vi "VNS Zobolas Local Search wOSSPClass.vi"(0 "OSSP_Problem.lvclass":refnum<class "OSSP_Problem.lvclass">, 1 "Max Allowed Time Passed?":bool, 3 "Reorder?":bool, 5 "Schedule In":u16[](array[numeric]), 7 "Scheduler":T1, 9 "Max Iteration Count":i32=1, 11 "error in (no error)":errorcluster, 12 "Number of Neighborhoods":i32=2, 14 "Objective":T2) -> (4 "OSSP_Problem out":refnum<class "OSSP_Problem.lvclass">, 6 "VNS Result Out":u16[](array[numeric]), 10 "Makespan/Tardiness(FIFO Engine)":u16, 15 "error out":errorcluster)   [LabVIEW 2013]
uses:
  Classes/OSSP_Problem.lvclass
  GA/Controls/Objective.ctl
  GA/Controls/Scheduler Type.ctl
  Classes/OSSP_Problem.lvclass/OSSP_Problem.ctl
  GA/SubVIS/Remove Duplicates In Array.vi
  Generate Two Indices for Local Search.vi
  Or-Opt(Zobolas) Neighborhood.vi
  Classes/Scheduler_Class/Prins FIFO Scheduler Methods and Controls/Methods/Calculate Makespan (Prins FIFO Engine).vi
  Classes/Scheduler_Class/Prins FIFO Scheduler Methods and Controls/Methods/Calculate Tardiness (Prins FIFO Engine).vi
  Classes/Scheduler_Class/NonDelay Scheduler/Non Delay Scheduler Engine.vi
  Classes/OSSP_Problem_Class/Getters/Read Number of Jobs.vi
  Classes/OSSP_Problem_Class/Getters/Read Processing Times.vi
  GA/SubVIS/Calcualte General Tardiness.vi
  Classes/OSSP_Problem_Class/Getters/Read Due Dates.vi
  Classes/Scheduler_Class/Giffler Thompson Active Schedule Engine.vi
  Classes/Scheduler_Class/Prins FIFO Scheduler Methods and Controls/Prins FIFO Scheduler.vi
  Classes/Scheduler_Class/Prins FIFO Scheduler Methods and Controls/Methods/Calculate Final Completion Times of Jobs.vi
  Classes/Scheduler_Class/Prins FIFO Scheduler Methods and Controls/Methods/Reorder Schedule(Prins FIFO) based on Start Times.vi
  Classes/Scheduler_Class/Operation to Machine Job Tuple.vi
  Classes/Scheduler_Class/Prins FIFO Scheduler Methods and Controls/Methods/UpdateMachineGaps.vi
  Classes/Scheduler_Class/Prins FIFO Scheduler Methods and Controls/Methods/UpdateJobGaps.vi
  Classes/Scheduler_Class/Prins FIFO Scheduler Methods and Controls/Methods/Find Intersecting Gaps.vi
  Classes/Scheduler_Class/GT Algorithm Find M_ok and J_ok.vi
  Classes/Scheduler_Class/Prins FIFO Scheduler Methods and Controls/Methods/Transform to Plain Job and Machine Gaps Array.vi
  Classes/Scheduler_Class/Semiactive Scheduler/Semi Active Scheduler Engine.vi
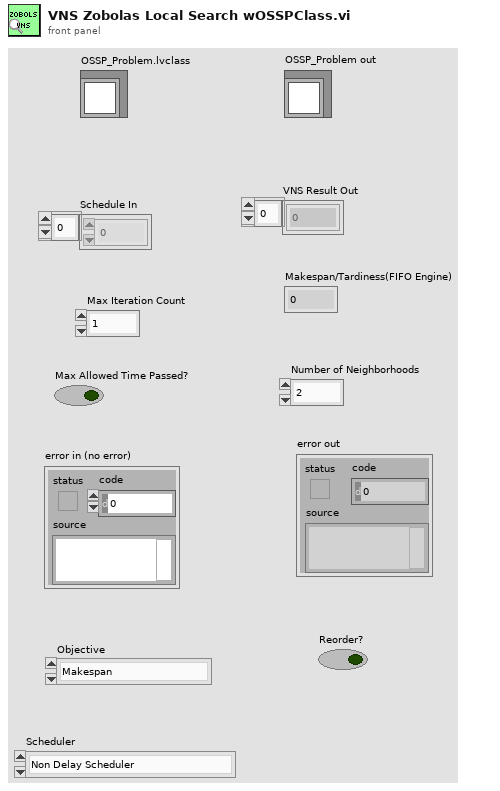
[diagram p1: front panel]
types:
  T1 = typedef "Scheduler Type.ctl" = enum16{"Non Delay Scheduler", "GT Active Scheduler", "My Faulty Scheduler", "Prins FIFO Scheduler", "SemiActive Scheduler"}
  T2 = typedef "Objective.ctl" = enum16{"Makespan", "Total Tardiness"}
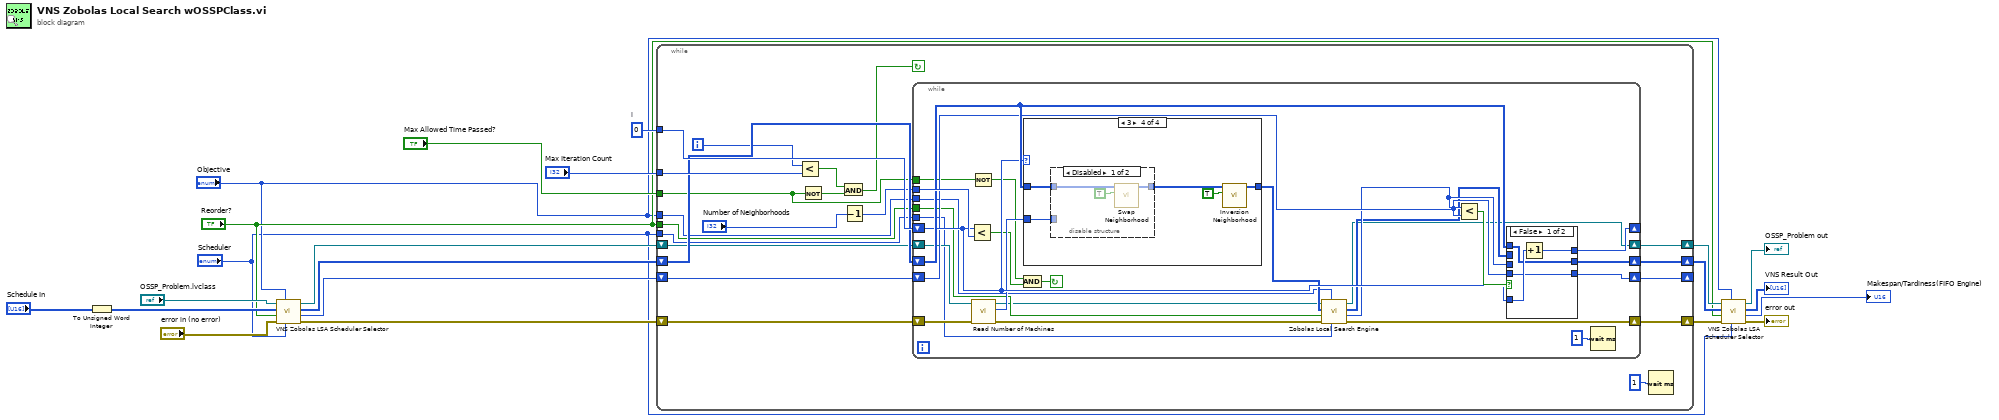
[diagram p0: block diagram]
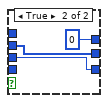
[diagram p2: hidden frame]
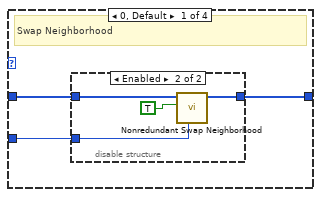
[diagram p3: hidden frame]
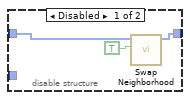
[diagram p4: hidden frame]
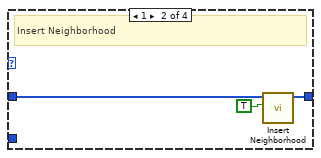
[diagram p5: hidden frame]
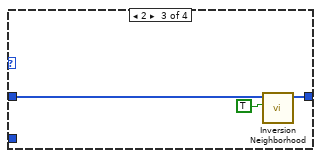
[diagram p6: hidden frame]
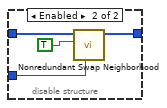
[diagram p7: hidden frame]
diagram:
  w20 = 0  # i
  n1 = To Unsigned Word Integer(number="Schedule In") -> (unsigned 16bit integer=w15:u16[])
  n2 = call "VNS Zobolas LSA Scheduler Selector.vi"("Scheduler"="Scheduler", "Objective"="Objective", "error in (no error)"="error in (no error)", "Reorder?"="Reorder?", "Schedule in"=w15, "OSSP_Problem in"="OSSP_Problem.lvclass") -> ("error out"=w14:errorcluster, "Total Tardiness (U16)"=w11:u16, "Schedule out"=w13:u16[], "OSSP_Problem out"=w12:refnum<class "OSSP_Problem.lvclass">)  [unwired: 2 in]
  n3 = while {
    tunnel: "Max Iteration Count" -> [w42]
    tunnel: w20 -> [w41]
    shift-right: [w40] -> w7
    shift-left: w13 -> [w39]
    shift-right: [w37] -> _
    shift-left: w11 -> [w38]
    shift-right: [w35] -> w8
    shift-left: w12 -> [w36]
    shift-right: [w33] -> w10
    shift-left: w14 -> [w34]
    tunnel: "Max Allowed Time Passed?" -> [w30]
    tunnel: "Objective" -> [w24]
    tunnel: "Reorder?" -> [w23]
    tunnel: "Scheduler" -> [w22]
    i -> [w31]
    stop <- w28 continue-if-true
    n4 = Less?(x=w31, y=w42) -> (x < y?=w32:bool)
    n5 = Not(x=w30) -> (.not. x?=w29:bool)
    n6 = And(x=w32, y=w29) -> (x .and. y?=w28:bool)
    n7 = Decrement(x="Number of Neighborhoods") -> (x-1=w25:i32)
    n8 = while {
      tunnel: w25 -> [w67]
      shift-right: [w66] -> _
      shift-left: w41 -> [w63]
      shift-right: [w65] -> w40
      shift-left: w39 -> [w64]
      shift-right: [w62] -> w37
      shift-left: w38 -> [w61]
      shift-right: [w51] -> w35
      shift-left: w36 -> [w48]
      shift-right: [w44] -> w33
      shift-left: w34 -> [w47]
      tunnel: w30 -> [w59]
      tunnel: w24 -> [w50]
      tunnel: w23 -> [w49]
      tunnel: w22 -> [w43]
      stop <- w56 continue-if-true
      n9 = Less?(x=w63, y=w67) -> (x < y?=w57:bool)
      n10 = Not(x=w59) -> (.not. x?=w58:bool)
      n11 = call "Read Number of Machines.vi"("error in (no error)"=w47, "OSSP_Problem in"=w48) -> ("error out"=w45:errorcluster, "Number of Machines"=w60:i32, "OSSP_Problem out"=w46:refnum<class "OSSP_Problem.lvclass">)  [unwired: 7 in]
      n12 = And(x=w58, y=w57) -> (x .and. y?=w56:bool)
      n13 = case shown="3" w63 {
        tunnel: w64 -> [w78 w88 w91 w96]
        tunnel: [w77 w87 w90 w94] -> w54
        tunnel: w60 -> [w76 _ _ w92]
        frame 0, Default {
          # "Swap Neighborhood"
          n14 = disable-structure shown="Enabled" {
            disable-tunnel: w78 -> [w81 w85]
            disable-tunnel: [w80 w84] -> w77
            disable-tunnel: w76 -> [_ w82]
            frame Disabled {
              n15 = call "Swap Neighborhood.vi"("Generate Random Indices?"=TRUE, "Schedule In"=w81) -> ("Schedule Out"=w80:u16[])  [unwired: 9 in]
            }
            frame Enabled {
              n16 = call "Nonredundant Swap Neighborhood.vi"("Number of Machines"=w82, "Generate Random indices?"=TRUE, "Schedule in"=w85) -> ("Schedule out"=w84:u16[])  [unwired: 8 in]
            }
          }
        }
        frame 1 {
          # "Insert Neighborhood"
          n17 = call "Insert Neighborhood.vi"("Generate Random Indices?"=TRUE, "C'"=w88) -> ("Chromosome Out"=w87:u16[])  [unwired: 9 in]
        }
        frame 2 {
          n18 = call "Inversion Neighborhood.vi"("Generate Random Indices?"=TRUE, "Schedule in"=w91) -> ("Schedule out"=w90:u16[])  [unwired: 9 in]
        }
        frame 3 {
          n19 = disable-structure shown="Disabled" {
            disable-tunnel: w96 -> [w99 w103]
            disable-tunnel: [w98 w102] -> w95
            disable-tunnel: w92 -> [_ w100]
            frame Disabled {
              n20 = call "Swap Neighborhood.vi"("Generate Random Indices?"=TRUE, "Schedule In"=w99) -> ("Schedule Out"=w98:u16[])  [unwired: 9 in]
            }
            frame Enabled {
              n21 = call "Nonredundant Swap Neighborhood.vi"("Number of Machines"=w100, "Generate Random indices?"=TRUE, "Schedule in"=w103) -> ("Schedule out"=w102:u16[])  [unwired: 8 in]
            }
          }
          n22 = call "Inversion Neighborhood.vi"("Generate Random Indices?"=TRUE, "Schedule in"=w95) -> ("Schedule out"=w94:u16[])  [unwired: 9 in]
        }
      }
      n23 = call "Zobolas Local Search Engine.vi"("Scheduler"=w43, "Objective"=w50, "error in (no error)"=w45, "Reorder?"=w49, "C'"=w54, "OSSP_Problem In"=w46) -> ("error out"=w44:errorcluster, "Tardiness of C\""=w53:u16, "C\""=w52:u16[], "OSSP_Problem out"=w51:refnum<class "OSSP_Problem.lvclass">)  [unwired: 2 in]
      n24 = Less?(x=w53, y=w61) -> (x < y?=w68:bool)
      n25 = case shown="False" w68 {
        tunnel: w63 -> [w71 _]
        tunnel: w52 -> [_ w74]
        tunnel: [w72 0] -> w66
        tunnel: [w70 w74] -> w65
        tunnel: w64 -> [w70 _]
        tunnel: w53 -> [_ w73]
        tunnel: [w69 w73] -> w62
        tunnel: w61 -> [w69 _]
        frame False {
          n26 = Increment(x=w71) -> (x+1=w72:i32)
        }
        frame True {
        }
      }
      n27 = Wait (ms)(milliseconds to wait=u32 1) -> ()  [unwired: 1 out]
    }
    n28 = Wait (ms)(milliseconds to wait=u32 1) -> ()  [unwired: 1 out]
  }
  n29 = call "VNS Zobolas LSA Scheduler Selector.vi"("Scheduler"="Scheduler", "Objective"="Objective", "error in (no error)"=w10, "Reorder?"="Reorder?", "Schedule in"=w7, "OSSP_Problem in"=w8) -> ("error out"=→"error out":errorcluster, "Total Tardiness (U16)"=→"Makespan/Tardiness(FIFO Engine)":u16, "Schedule out"=→"VNS Result Out":u16[], "OSSP_Problem out"=→"OSSP_Problem out":refnum<class "OSSP_Problem.lvclass">)  [unwired: 2 in]
